vi "Split the Difference.vi"(10 "Y":i16, 11 "X":i16) -> (3 "Half the Difference":dbl)   [LabVIEW 2020]
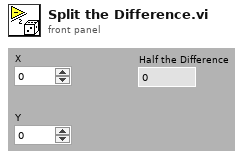
[diagram p1: front panel]
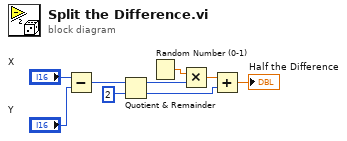
[diagram p0: block diagram]
diagram:
  n1 = Subtract(x="X", y="Y") -> (x-y=w3:i16)
  n2 = Quotient & Remainder(x=w3, y=i16 2) -> (x-y*floor(x/y)=w5:i16, floor(x/y)=w8:i16)
  n3 = Random Number (0-1)() -> (number: 0 to 1=w6:dbl)
  n4 = Multiply(x=w6, y=w5) -> (x*y=w7:dbl)
  n5 = Add(x=w7, y=w8) -> (x+y=→"Half the Difference":dbl)
